vi "niFPGA Saturate.vi"(0 "upper limit":i32=1073741823, 2 "input":i32, 3 "lower limit":i32=-1073741824) -> (7 "output":i32)   [LabVIEW 2020]
doc: "Limits the valid range of a signal to that specified by <B>Upper limit</B> and <B>Lower limit</B>. You can configure the VI to specify the integer or bit limits and signed or unsigned inputs."
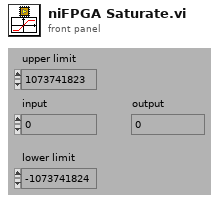
[diagram p1: front panel]
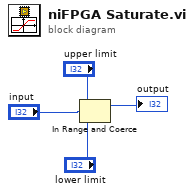
[diagram p0: block diagram]
diagram:
  n1 = In Range and Coerce(upper limit="upper limit", x="input", lower limit="lower limit") -> (coerced(x)=→"output":i32)  [unwired: 1 out]
